vi "host.bats.parser.tester.vi"() -> ()   [LabVIEW 2020]
uses:
  <vilib>/rvi/interface/RandomDataEmulation/nirviRandomDataOpen.vi
  <vilib>/rvi/interface/common/niFpgaCacheSessionInfoDynamic.vi
  <vilib>/Utility/error.llb/Error Cluster From Error Code.vi
  <vilib>/rvi/errors/niLvFpgaAdjustHostInterfaceError.vi
  <vilib>/FPGAPlugInAG/Dynamic/niLvFpga_Close_Dynamic.vi
  <vilib>/rvi/interface/nirviOpenFPGA/nirviOpenFPGA.xnode
  arty/test/fpga.bats.parser.test.harness.vi
  <vilib>/rvi/interface/nirviMethod/nirviMethod.xnode
  <vilib>/rvi/interface/nirviCloseFPGA/nirviCloseFPGA.xnode
  <vilib>/rvi/errors/niLvFpgaMergeErrorWithErrorCode.vi
  <vilib>/FPGAPlugInAG/Dynamic/niLvFpga_ReadFifo_Dynamic.vi
  <vilib>/FPGAPlugInAG/Dynamic/niLvFpga_WriteFifo_Dynamic.vi
panel:
  in  "Execute?":bool
  in  "Raw File":string="raw.pitch.dat"
  in  "Use Raw File":bool=TRUE
  in  "Raw String":string
  out "data string":string
  out "Data":u8[](array[numeric]) format="%.0x"
  out "error out":errorcluster
  in  "error in":errorcluster
  out "Data toSend":u16[](array[numeric])=[0, 10, 53, 0, 1, 2, 96, 164, 76, 99, 247, 234, 8, 0, 69, 0, 0, 90, 203, 42, 0, 0, 128, 17, 235, 17, 192, 168, 1, 202, 192, 168, 1, 60, 251, 70, 23, 113, 0, 70, 25, 65, 84, 104, 105, 115, 32, 105, 115, 32, 116, 104, 101, 32, 109, 101, 115, 115, 97, 103, 101, 46, 32, 73, 116, 32, 119, 105, 108, 108, 32, 98, 101, 32, 114, 101, 112, 101, 97, 116, 101, 100, 46, 32, 32, 84, 111, 32, 71, 101, 110, 101, 115, 121, 115, 32, 111, 114, 32, 65, 114, 116, 121, 46, 37, 126, 148, 412] format="%.0x"
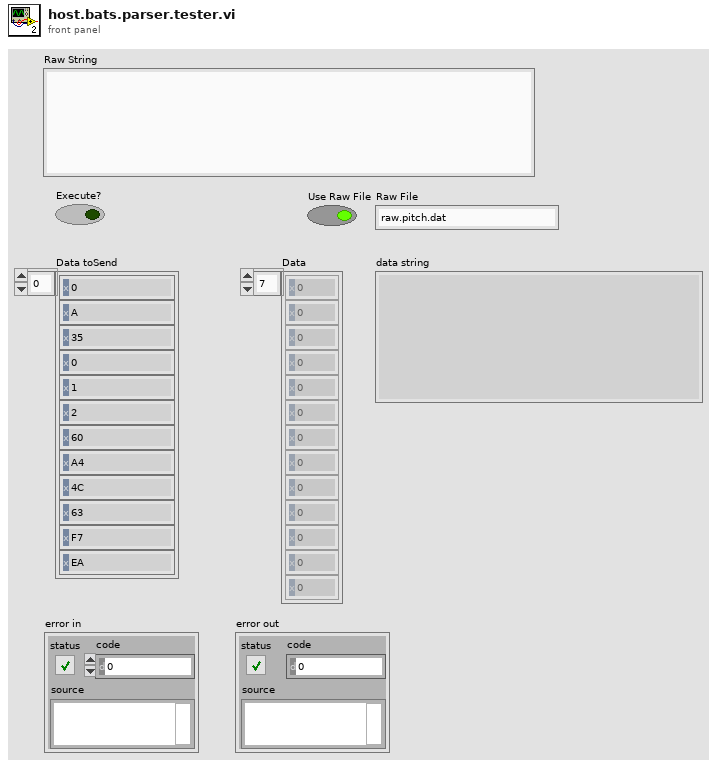
[diagram p1: front panel]
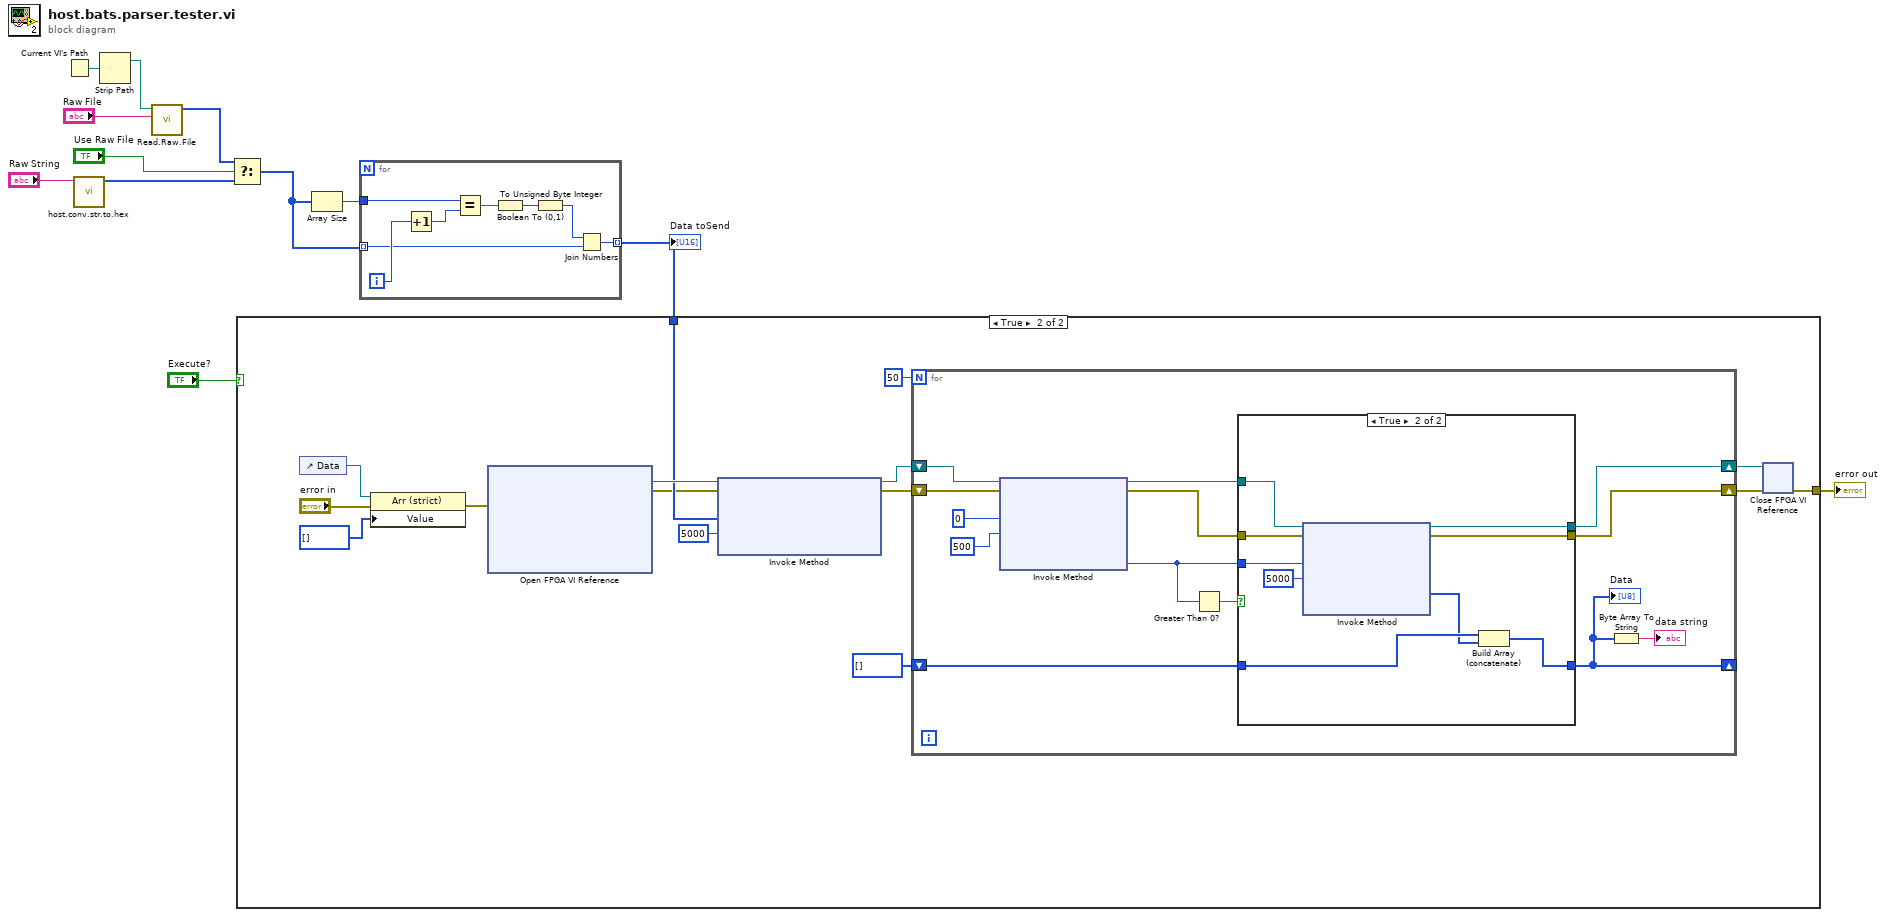
[diagram p0: block diagram]
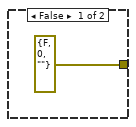
[diagram p2: hidden frame]
diagram:
  n1 = Current VI's Path() -> (path=w7:path)
  n2 = call "host.conv.str.to.hex.vi"("String"="Raw String") -> ("Array 2"=w8:u8[])  [unwired: 10 in]
  n3 = Strip Path(path=w7) -> (stripped path=w5:path)  [unwired: 1 out]
  n4 = call "Read.Raw.File.vi"("Raw File"="Raw File", "Path"=w5) -> ("data"=w2:u8[])  [unwired: 9 in]
  n5 = Select(t=w2, s="Use Raw File", f=w8) -> (s? t:f=w4:u8[])
  n6 = Array Size(array=w4) -> (size(s)=w12:i32)
  n7 = for {
    tunnel: w4 -> [w18] mode=indexing
    tunnel: w12 -> [w20]
    tunnel: [w14] -> w11 mode=indexing
    i -> [w19]
    n8 = Increment(x=w19) -> (x+1=w13:i32)
    n9 = Equal?(x=w20, y=w13) -> (x = y?=w17:bool)
    n10 = Boolean To (0,1)(Boolean=w17) -> (0, 1=w16:i16)
    n11 = To Unsigned Byte Integer(number=w16) -> (unsigned 8bit integer=w15:u8)
    n12 = Join Numbers(hi=w15, lo=w18) -> ((hi.lo)=w14:u16)
  }
  "Data toSend" <- w11
  n13 = case shown="True" "Execute?" {
    tunnel: w11 -> [_ w35]
    tunnel: [errorcluster {"status"=FALSE, "code"=0, "source"=""} ("error out") w33] -> w10
    frame False {
    }
    frame True {
      n14 = control-ref of="Data"() -> (w26:refnum<vi>)
      n15 = property class="Arr (strict)"(reference=w26, error in="error in", "Value"=u8[] []) -> (error out=w23:errorcluster)  [unwired: 1 out]
      n16 = xnode "Open FPGA VI Reference"("error in"=w23) -> ("FPGA VI Reference Out"=w36:refnum<k20>, "error out"=w22:errorcluster)  [unwired: 1 in]
      n17 = xnode "Invoke Method"("FPGA VI Reference In"=w36, "error in"=w22, "Data"=w35, "Timeout (ms)"=5000) -> ("FPGA VI Reference Out"=w32:refnum<k20>, "error out"=w31:errorcluster)  [unwired: 1 out]
      n18 = for {
        N: 50 -> [_]
        shift-right: [w38] -> _
        shift-left: u8[] [] ("Data") -> [w42]
        shift-right: [w41] -> w28
        shift-left: w32 -> [w49]
        shift-right: [w40] -> w27
        shift-left: w31 -> [w48]
        n19 = xnode "Invoke Method"("FPGA VI Reference In"=w49, "error in"=w48, "Number of Elements"=u32 0, "Timeout (ms)"=500) -> ("FPGA VI Reference Out"=w43:refnum<k20>, "error out"=w39:errorcluster, "Elements Remaining"=w44:u32)  [unwired: 1 out]
        n20 = Greater Than 0?(x=w44) -> (x > 0?=w45:bool)
        n21 = case shown="True" w45 {
          tunnel: w44 -> [_ w61]
          tunnel: w43 -> [w51 w59]
          tunnel: [w52 w56] -> w38
          tunnel: w42 -> [w52 w58]
          tunnel: [w51 w55] -> w41
          tunnel: [w50 w54] -> w40
          tunnel: w39 -> [w50 w53]
          frame False {
          }
          frame True {
            n22 = xnode "Invoke Method"("FPGA VI Reference In"=w59, "error in"=w53, "Number of Elements"=w61, "Timeout (ms)"=5000) -> ("FPGA VI Reference Out"=w55:refnum<k20>, "error out"=w54:errorcluster, "Data"=w57:u8[])  [unwired: 1 out]
            n23 = Build Array (concatenate)(w58, w57) -> (w56:u8[])
          }
        }
        "Data" <- w38
        n24 = Byte Array To String(unsigned byte array=w38) -> (string=→"data string":string)
      }
      n25 = xnode "Close FPGA VI Reference"("FPGA VI Reference In"=w28, "error in"=w27) -> ("error out"=w33:errorcluster)
    }
  }
  "error out" <- w10
